vi "Create Plugin Configuration.vi"(6 "plugin timing":T1={"Decimation"=1, "Offset"=0}, 8 "channel count per transfer":i32, 9 "transfers per group":i32, 10 "group configs":cluster{"direction":T2, "timing":T1}[](array[cluster]), 11 "plugin class":string) -> (3 "plugin configuration":T3)   [LabVIEW 2017]
uses:
  DSF.Shared.Refactor.Typedefs.Plugin Configuration.Aggregate.ctl
  DSF.Shared.Typedefs.Cycle Timing Factors.ctl
  DSF.Shared.Refactor.Typedefs.Transfer Group Configuration.Aggregate.ctl
  DSF.Shared.Typedefs.Direction.ctl
  DSF.Shared.Refactor.Typedefs.Transfer Configuration.ctl
  DSF.Shared.Typedefs.Byte Order.ctl
  DSF.Shared.Refactor.Typedefs.Channel Array Configuration.ctl
  DSF.Shared.Typedefs.Data Type.ctl
  DSF.Shared.lvlib
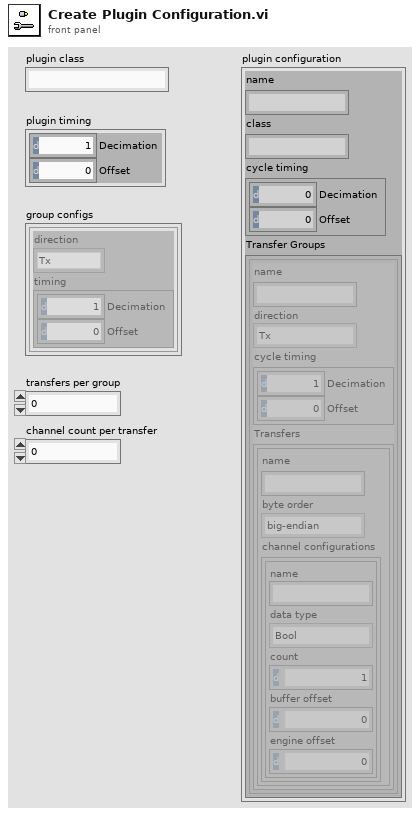
[diagram p1: front panel]
types:
  T1 = typedef "DSF.Shared.lvlib/DSF.Shared.Typedefs.Cycle Timing Factors.ctl" = cluster{"Decimation":u64, "Offset":u64}
  T2 = typedef "DSF.Shared.lvlib/DSF.Shared.Typedefs.Direction.ctl" = enum8{"Tx", "Rx"}
  T3 = typedef "DSF.Shared.lvlib/DSF.Shared.Refactor.Typedefs.Plugin Configuration.Aggregate.ctl" = cluster{"name":string, "class":string, "cycle timing":T1, "Transfer Groups":T4[]}
  T4 = typedef "DSF.Shared.lvlib/DSF.Shared.Refactor.Typedefs.Transfer Group Configuration.Aggregate.ctl" = cluster{"name":string, "direction":T2, "cycle timing":T1, "Transfers":T5[]}
  T5 = typedef "DSF.Shared.lvlib/DSF.Shared.Refactor.Typedefs.Transfer Configuration.ctl" = cluster{"name":string, "byte order":T6, "channel configurations":T7[]}
  T6 = typedef "DSF.Shared.lvlib/DSF.Shared.Typedefs.Byte Order.ctl" = enum8{"big-endian", "little-endian"}
  T7 = typedef "DSF.Shared.lvlib/DSF.Shared.Refactor.Typedefs.Channel Array Configuration.ctl" = cluster{"name":string, "data type":T8, "count":u64, "buffer offset":u64, "engine offset":u64}
  T8 = typedef "DSF.Shared.lvlib/DSF.Shared.Typedefs.Data Type.ctl" = enum8{"Bool", "SGL", "DBL", "I8", "I16", "I32", "I64", "U8", "U16", "U32", "U64"}
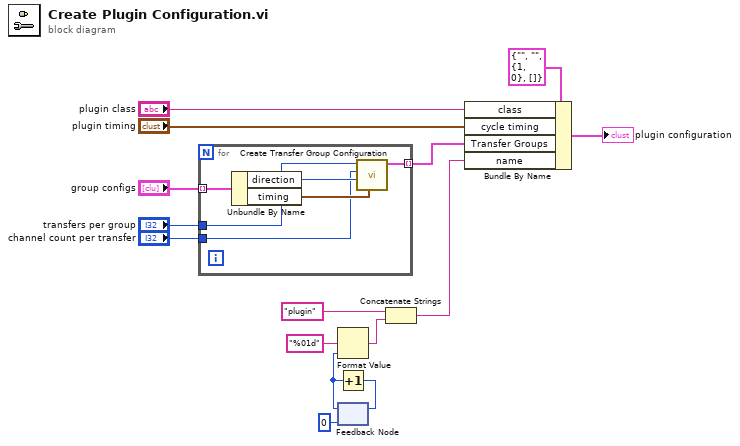
[diagram p0: block diagram]
diagram:
  n1 = for {
    tunnel: "transfers per group" -> [w20]
    tunnel: [w21] -> w8 mode=indexing
    tunnel: "group configs" -> [w17] mode=indexing
    tunnel: "channel count per transfer" -> [w16]
    n2 = Unbundle By Name(w17) -> ("direction"=w19:T2, "timing"=w18:T1)
    n3 = call "Create Transfer Group Configuration.vi"("group timing (dec:1, off: 0)"=w18, "direction"=w19, "channel count per transfer"=w16, "transfers per group"=w20) -> ("transfer group"=w21:T4)  [unwired: 7 in]
  }
  n4 = feedback #1(0) -> (w13:i32)
  n5 = Format Value(format string="%01d", value (0)=w13) -> (output string=w10:string)  [unwired: 1 in]
  n6 = Increment(x=w13) -> (x+1=w14:i32)
  n7 = feedback-in #1(w14) -> ()
  n8 = Concatenate Strings("plugin" ("name"), w10) -> (w5:string)
  n9 = Bundle By Name(cluster=T3 {"name"="", "class"="", "cycle timing"={"Decimation"=1, "Offset"=0}, "Transfer Groups"=[]} ("Plugin Configuration"), "class"="plugin class", "cycle timing"="plugin timing", "Transfer Groups"=w8, "name"=w5) -> (→"plugin configuration":T3)
